vi "Main.vi"() -> ()   [LabVIEW 2016]
uses:
  <vilib>/picture/picture.llb/imagedata.ctl
panel:
  out "nInterfaceNum":u32
  in  "Path":path
  in  "SavePic":bool
  in  "pConvertInfo In 2":T1
  out "frameHandle":i64
  in  "DeviceInterfaceType":u16(ring) items=["GigE", "U3v", "CameraLink", "CXP"]
  in  "ExposureAuto":i32(ring)
  out "QuitFlag":bool
  in  "pConvertInfo In":T1
  in  "image data":T2 caption="图像数据"
  in  "Rectangle":T3
  in  "DeviceScanType":i32(ring)
  out "InterfaceOpened":bool
  out "hDev":i64
  out "hIFDev":i64
  out "interfaceKeyList":string[](array[string])
  out "HasInterface":bool
  out "Picture":picture
  out "Acquired Frames/s":dbl
  out "Processed Frames/s":dbl
  in  "TriggerSource":i32(ring)
  in  "ExecuteSoftTrig":bool
  in  "CloseTrig":bool
  in  "OpenTrig":bool
  in  "Stop":bool
  in  "Play":bool
  in  "Quit":bool
  in  "Height":i32
  in  "Width":i32
  in  "PixelFormat":i32(ring)
  in  "GainRaw":dbl
  in  "ExposureTime":dbl
  out "IsGrabbing":bool
  out "TrigModeOn":bool
  out "error out":errorcluster
  in  "error in":errorcluster
  in  "Close":bool
  in  "Open":bool
  out "HasDevices":bool
  in  "DeviceOpened":bool
  in  "DeviceList":i64(ring)
  in  "Discovery":bool
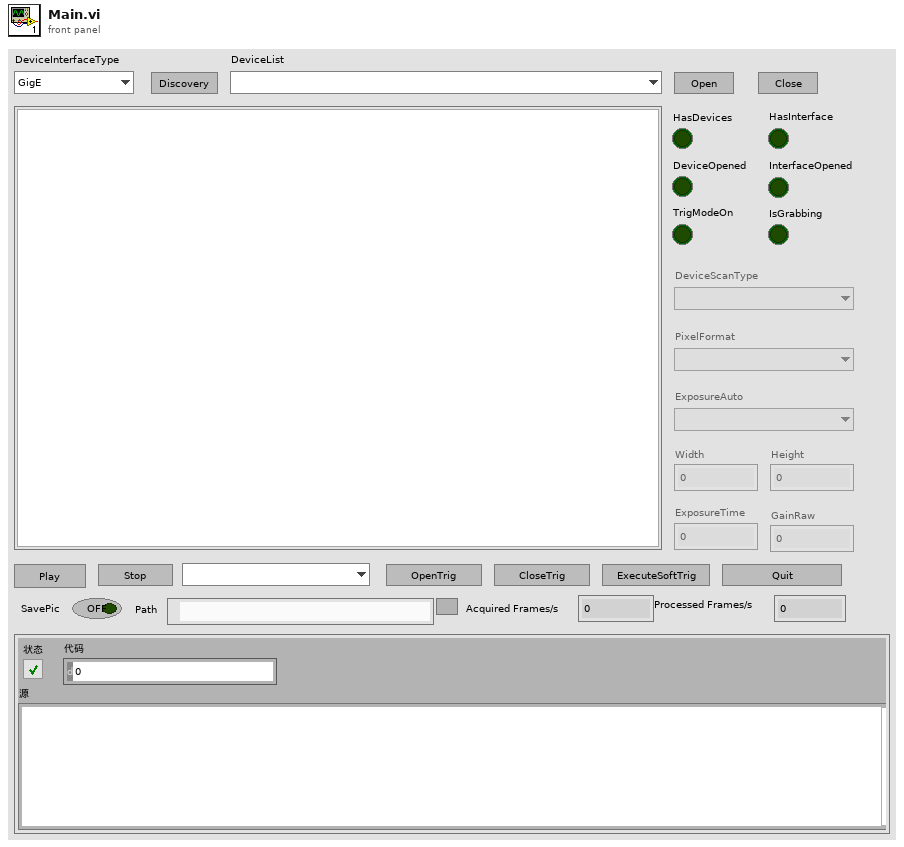
[diagram p1: front panel]
types:
  T1 = cluster{"nWidth":u32, "nHeight":u32, "enSrcPixelType":u32, "nSrcDataLen":u32, "nPaddingX":u32, "nPaddingY":u32, "eBayerDemosaic":u32, "eDstPixelFormat":u32, "nDstBufSize":u32, "nDstDataLen":u32, "nReserved0":u32, "nReserved1":u32, "nReserved2":u32, "nReserved3":u32, "nReserved4":u32, "nReserved5":u32, "nReserved6":u32, "nReserved7":u32}
  T2 = typedef "imagedata.ctl" = cluster{"image type":i32, "image depth":i32, "image":u8[], "mask":u8[], "colors":u32[], "Rectangle":cluster{"left":i16, "top":i16, "right":i16, "bottom":i16}}
  T3 = cluster{"left":i16, "top":i16, "right":i16, "bottom":i16}
  T4 = cluster{"blockId":u64, "status":u32, "width":u32, "height":u32, "size":u32, "pixelFormat":u32, "timeStamp":u64, "chunkCount":u32, "paddingX":u32, "paddingY":u32, "recvFrameTime":u32}
  T5 = cluster{"blockId":u64, "status":u32, "width":u32, "height":u32, "size":u32, "pixelFormat":i32, "timeStamp":u64, "chunkCount":u32, "paddingX":u32, "paddingY":u32, "recvFrameTime":u32}
  T6 = enum8{"Enabled", "Disabled", "Disabled and Grayed Out"}
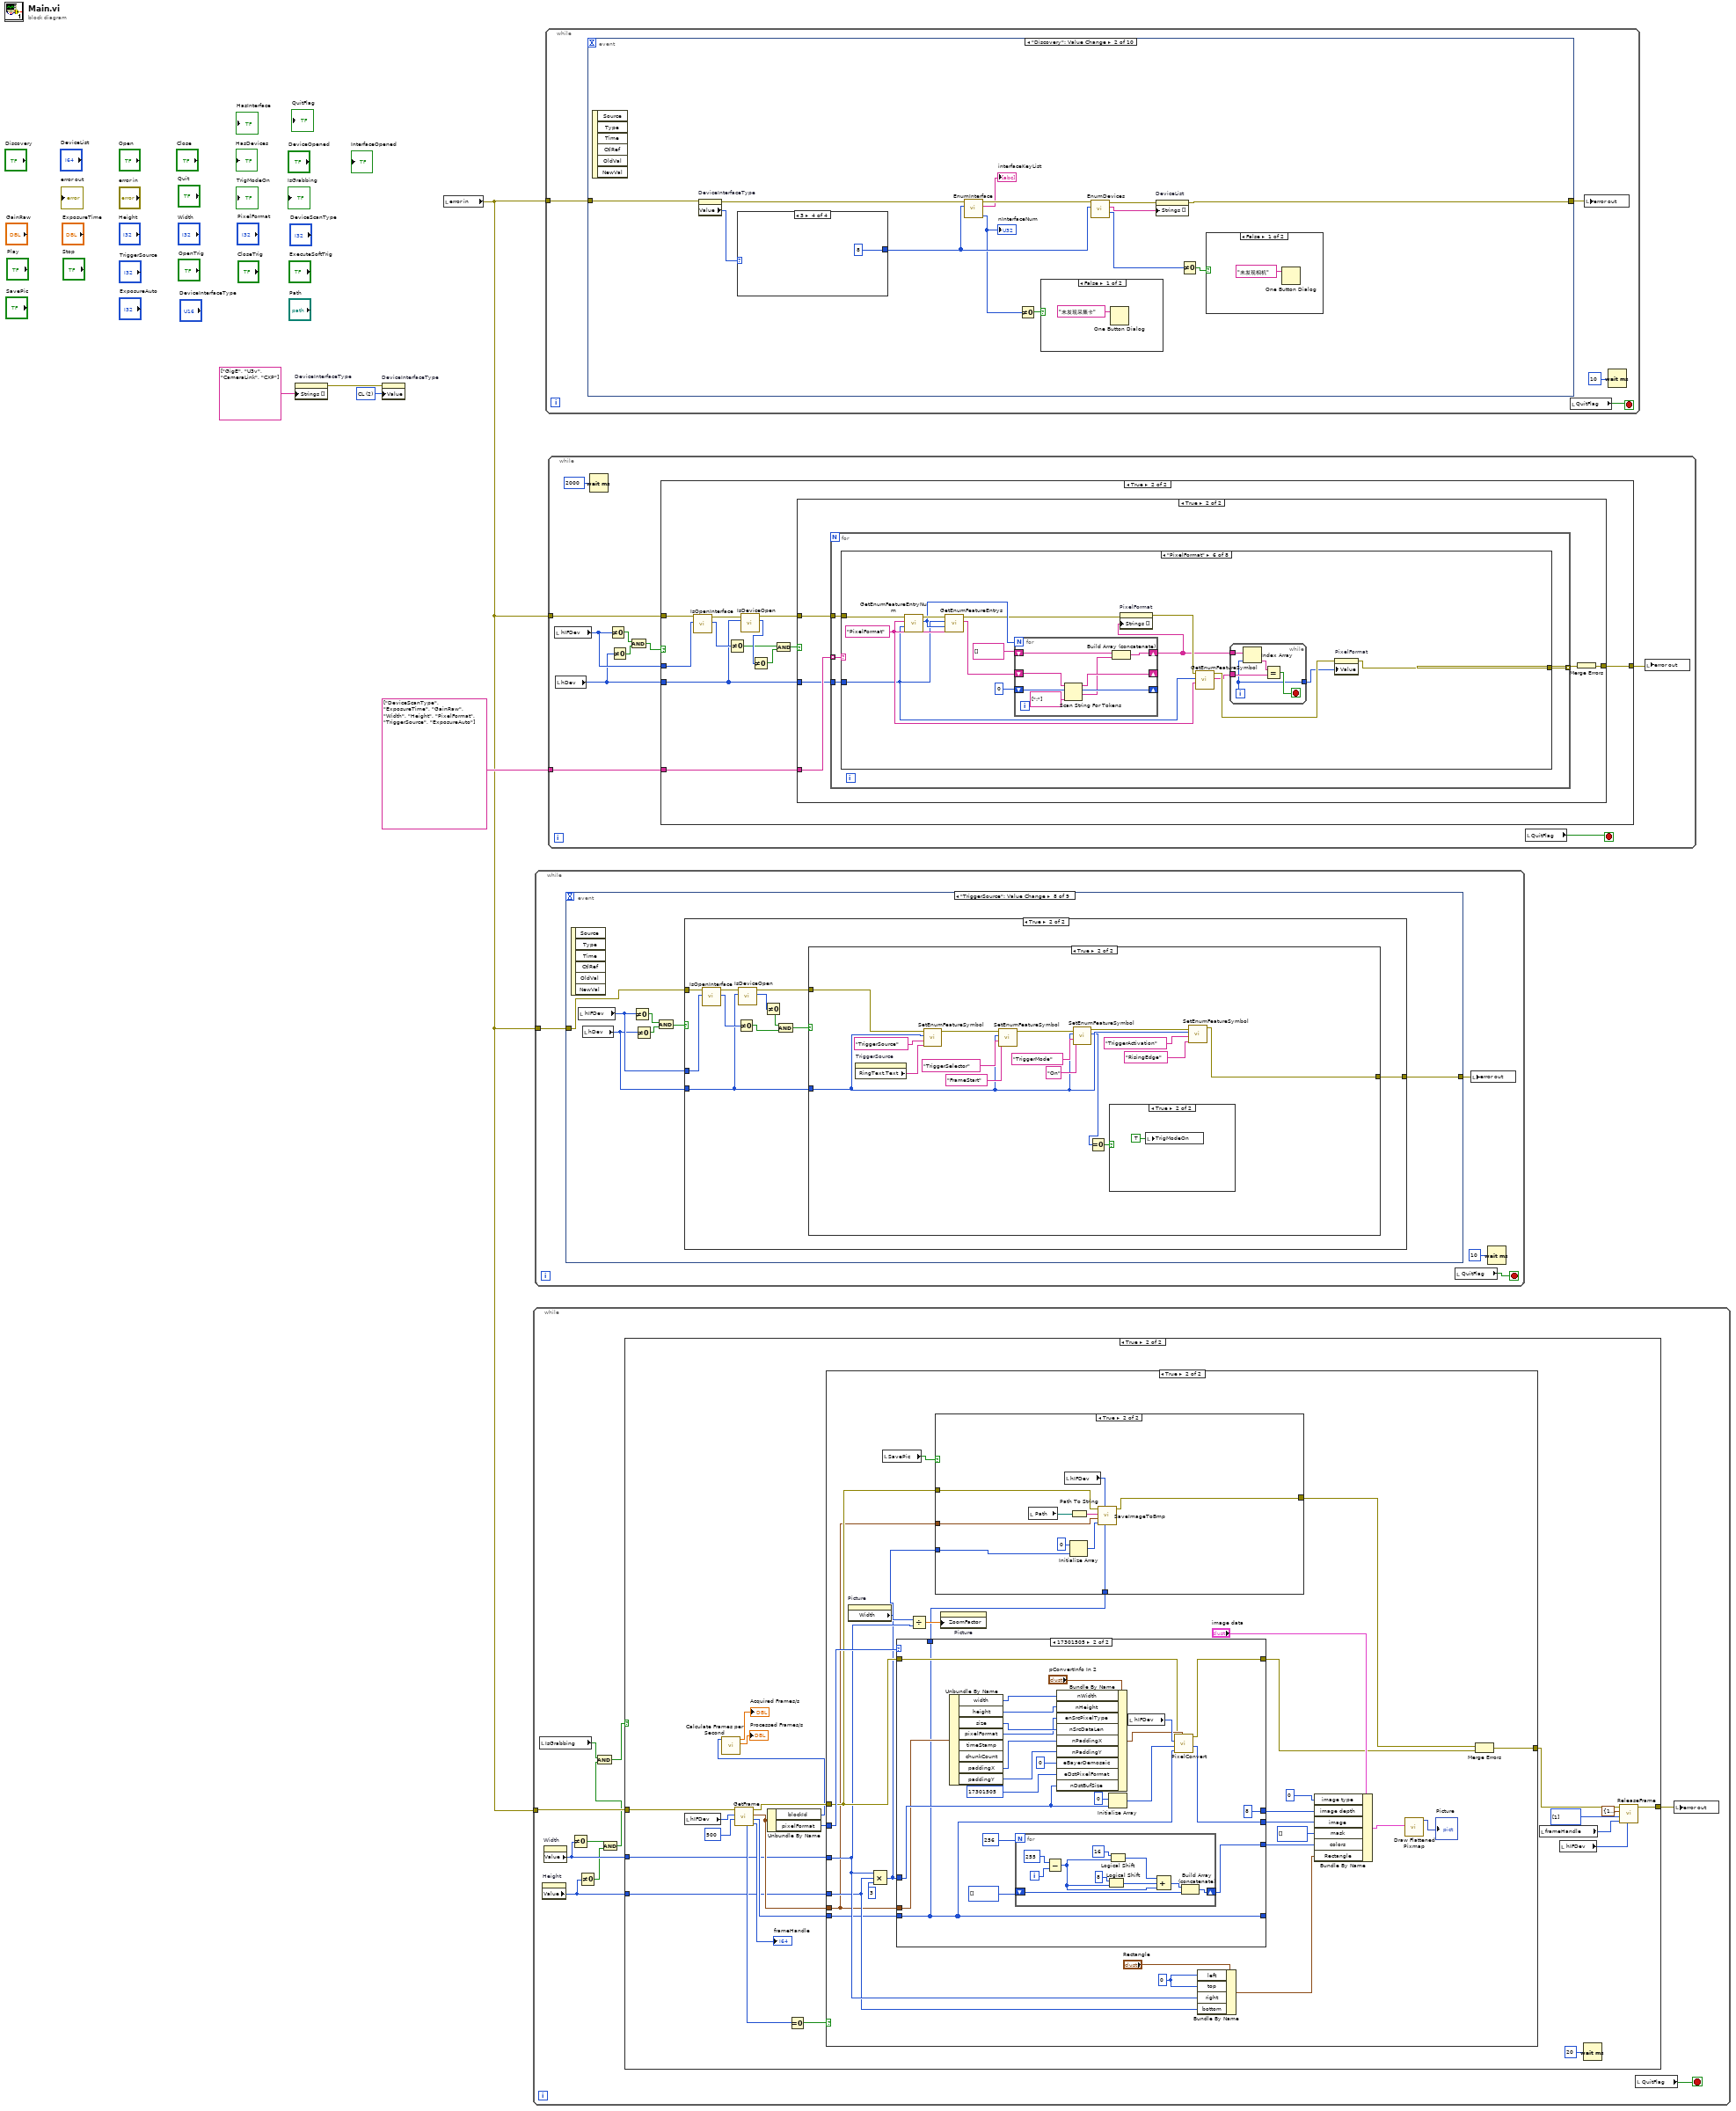
[diagram p0: block diagram]
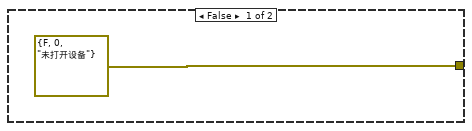
[diagram p2: hidden frame]
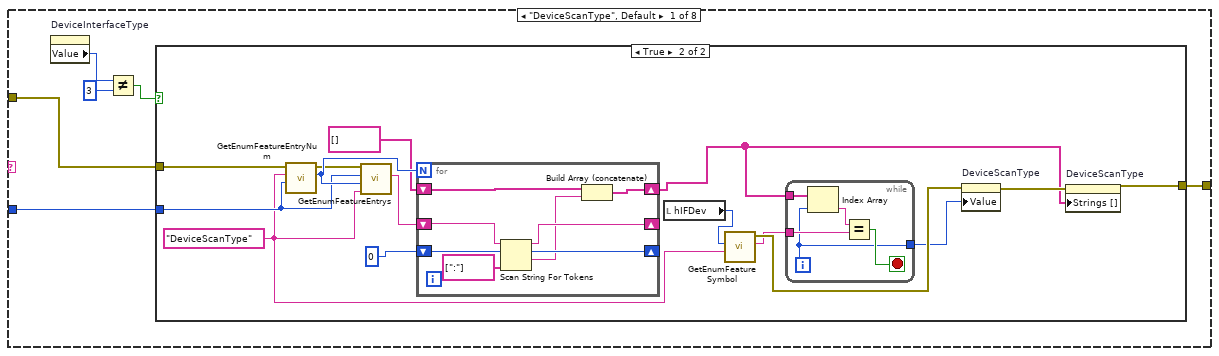
[diagram p4: hidden frame]
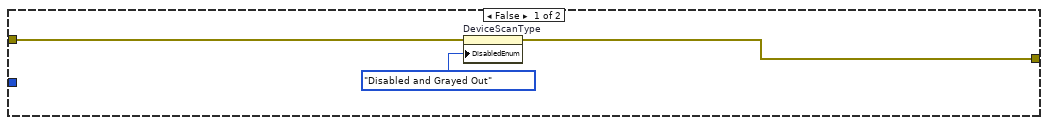
[diagram p5: hidden frame]
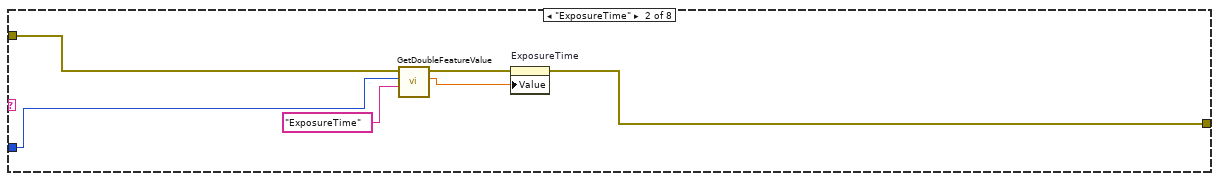
[diagram p6: hidden frame]
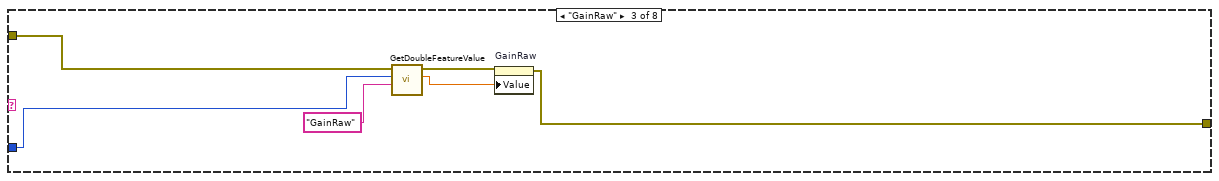
[diagram p7: hidden frame]
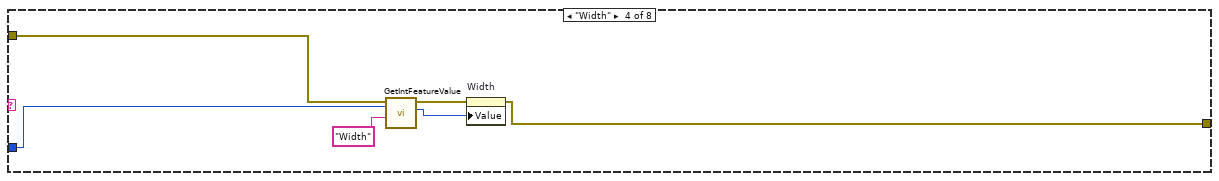
[diagram p8: hidden frame]
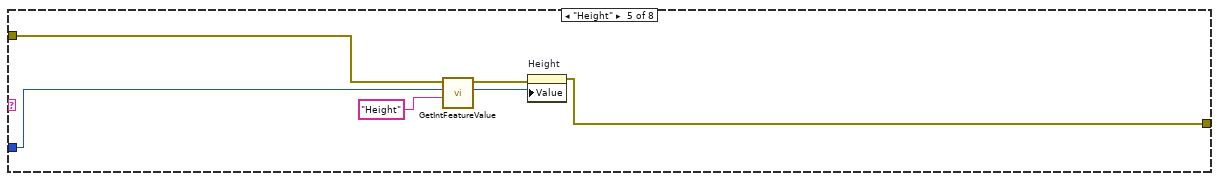
[diagram p9: hidden frame]
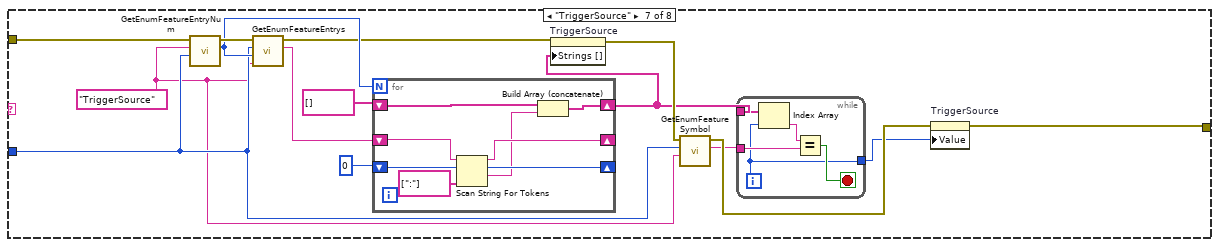
[diagram p10: hidden frame]
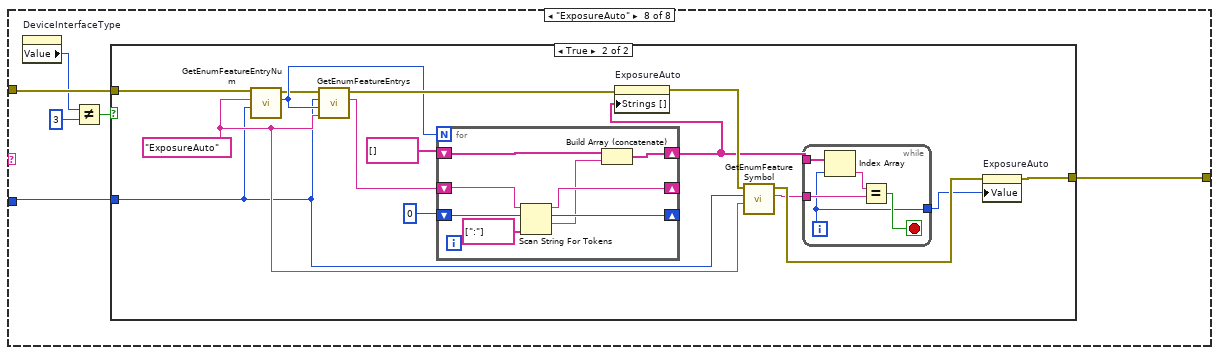
[diagram p11: hidden frame]
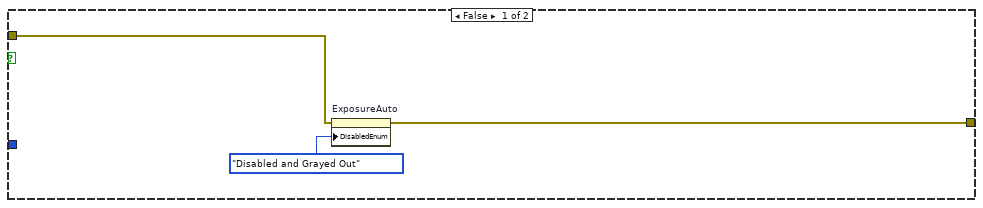
[diagram p12: hidden frame]
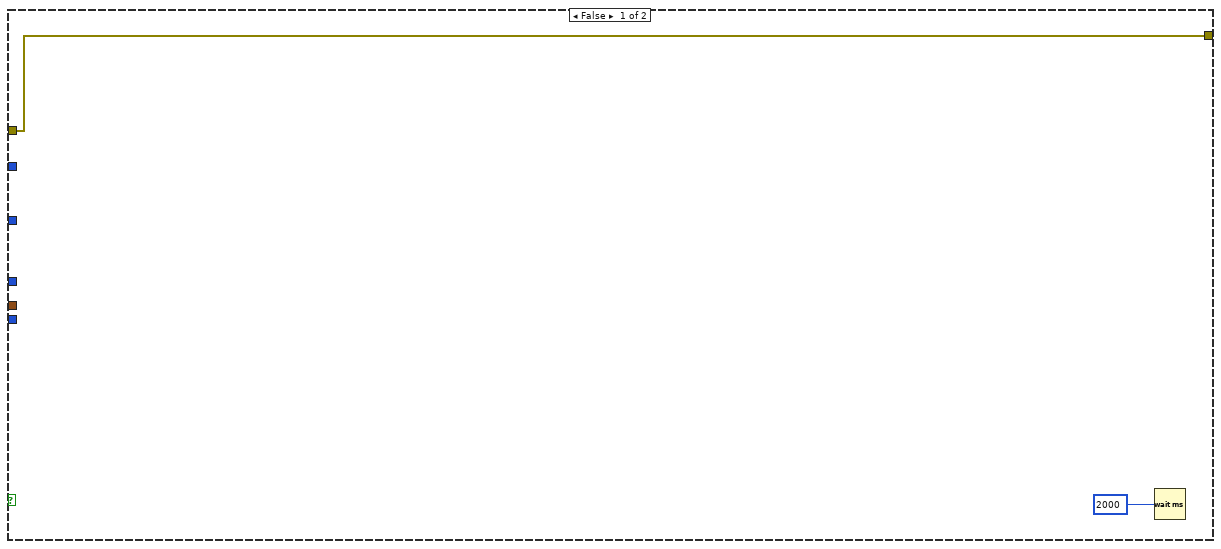
[diagram p14: hidden frame]
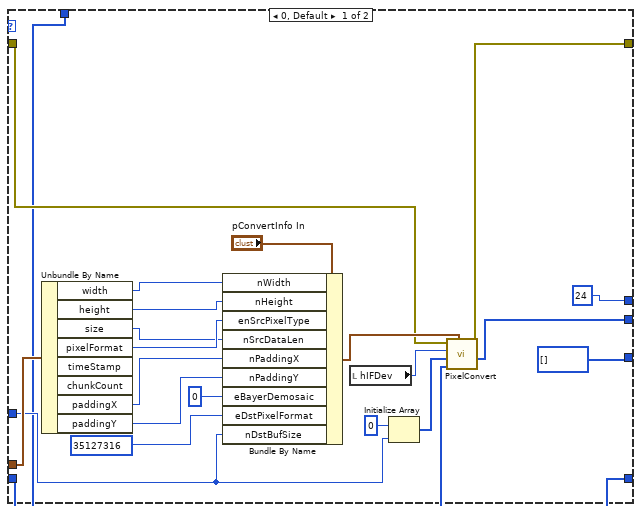
[diagram p16: hidden frame]
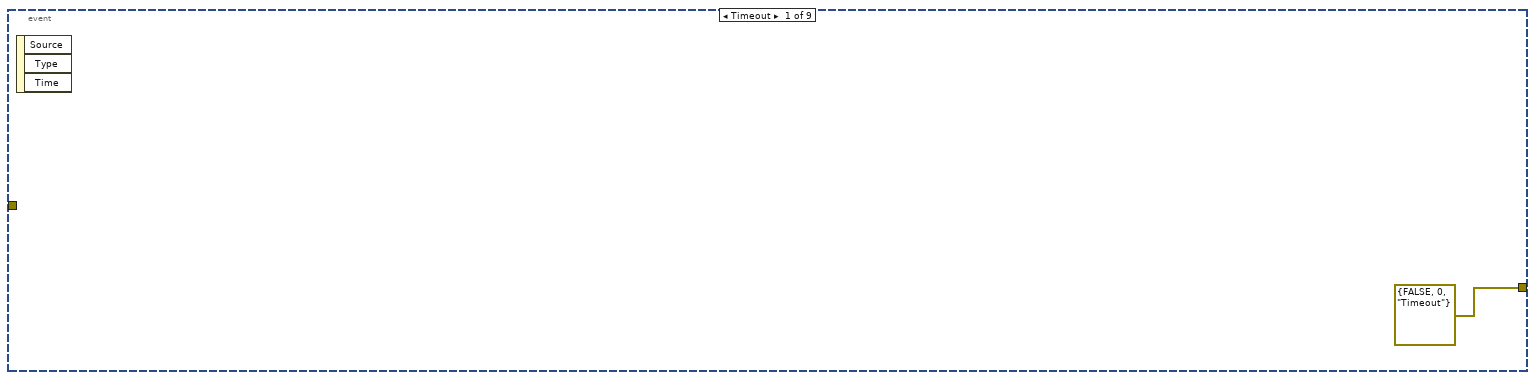
[diagram p17: hidden frame]
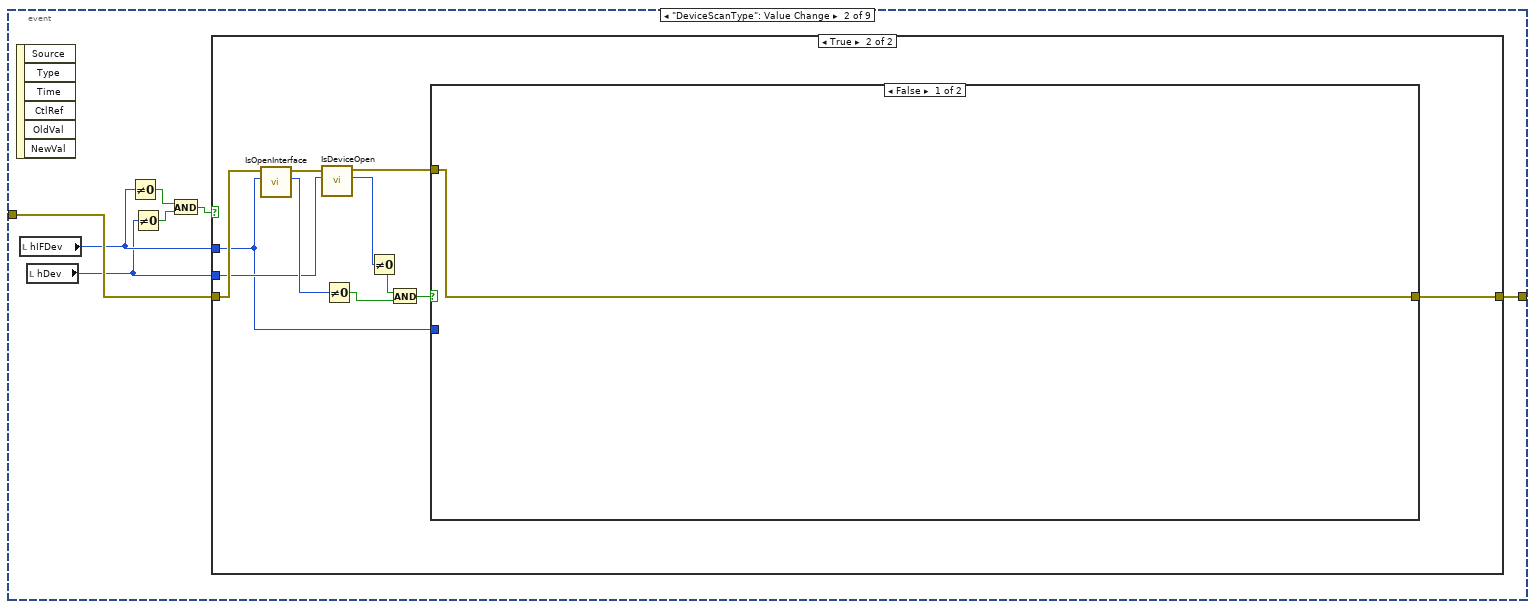
[diagram p18: hidden frame]
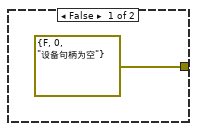
[diagram p19: hidden frame]
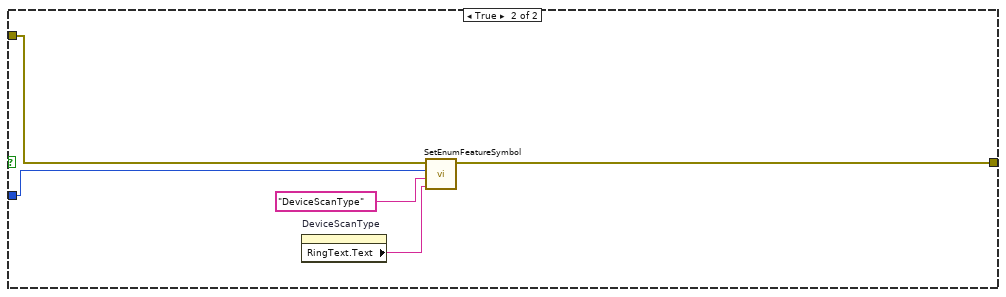
[diagram p20: hidden frame]
diagram:
  w2 = u16 2 items=["GigE", "U3v", "CL", "CXP"] ("DeviceInterfaceType")
  n1 = property on="DeviceInterfaceType" class="Ring (strict)"("Strings []"=string[] ["GigE", "U3v", "CameraLink", "CXP"]) -> (error out=w1:errorcluster)  [unwired: 2 in, 1 out]
  n2 = property on="DeviceInterfaceType" class="Ring (strict)"(error in=w1, "Value"=w2) -> ()  [unwired: 1 in, 2 out]
  n3 = local read "error in"() -> (w4:errorcluster)
  n4 = while {
    tunnel: w4 -> [w15]
    stop <- w13 stop-if-true
    n5 = local read "IsGrabbing"() -> (w8:bool)
    n6 = property on="Height" class="DigNum (strict)"() -> ("Value"=w10:i32)  [unwired: 2 in, 2 out]
    n7 = property on="Width" class="DigNum (strict)"() -> ("Value"=w11:i32)  [unwired: 2 in, 2 out]
    n8 = Not Equal To 0?(x=w11) -> (x != 0?=w12:bool)
    n9 = Not Equal To 0?(x=w10) -> (x != 0?=w9:bool)
    n10 = And(x=w12, y=w9) -> (x .and. y?=w7:bool)
    n11 = And(x=w8, y=w7) -> (x .and. y?=w6:bool)
    n12 = case shown="True" w6 {
      tunnel: w15 -> [w16 w24]
      tunnel: [w16 w28] -> w14
      tunnel: w11 -> [_ w20]
      tunnel: w10 -> [_ w19]
      frame False {
      }
      frame True {
        n13 = local read "hIFDev"() -> (w22:i64)
        n14 = call "GetFrame.vi"("timeoutMS"=u32 500, "handle"=w22, "error in (no error)"=w24) -> ("frameHandle"=→"frameHandle":i64, "pData"=w35:u8[], "pLbFrame out"=w36:T5, "error out"=w30:errorcluster, "return type"=w38:i32)  [unwired: 4 in]
        n15 = Unbundle By Name(w36) -> ("blockId"=w27:u64, "pixelFormat"=w31:i32)
        n16 = call <vilib>:"Calculate Frames per Second.vi"("Buffer Number"=w27) -> ("Processed Frames/s"=→"Processed Frames/s":dbl, "Acquired Frames/s"=→"Acquired Frames/s":dbl)  [unwired: 8 in, 1 out]
        n17 = Equal To 0?(x=w38) -> (x = 0?=w37:bool)
        n18 = case shown="True" w37 {
          tunnel: w36 -> [_ w45]
          tunnel: w35 -> [_ w43]
          tunnel: w20 -> [_ w47]
          tunnel: w19 -> [_ w46]
          tunnel: w31 -> [_ w63]
          tunnel: w30 -> [w40 w52]
          tunnel: [w40 w49] -> w29
          frame False {
            n19 = Wait (ms)(milliseconds to wait=u32 2000 ("等待时间（毫秒）")) -> ()  [unwired: 1 out]
          }
          frame True {
            w61 = i16 0 ("left")
            n20 = property on="Picture" class="Pict"() -> ("Width"=w65:u32)  [unwired: 2 in, 2 out]
            n21 = Compound Arithmetic op=MULTIPLY(w47, w46, 3) -> (w44:i32)
            n22 = local read "SavePic"() -> (w42:bool)
            n23 = case shown="17301505" w63 {
              tunnel: [i32[] [] w119] -> w56
              tunnel: w43 -> [w78 w99]
              tunnel: [w78 w99] -> _
              tunnel: [w86 w100] -> w53
              tunnel: [24 8] -> w54
              tunnel: w45 -> [w81 w106]
              tunnel: w52 -> [w83 w102]
              tunnel: [w82 w101] -> w50
              tunnel: w44 -> [w80 w107]
              tunnel: [w78 w99] -> w41
              frame 0, Default {
                n24 = Unbundle By Name(w81) -> ("width"=w97:u32, "height"=w96:u32, "size"=w79:u32, "pixelFormat"=w95:i32, "paddingX"=w94:u32, "paddingY"=w93:u32)  [unwired: 2 out]
                n25 = Bundle By Name(cluster="pConvertInfo In", "nWidth"=w97, "nHeight"=w96, "enSrcPixelType"=w95, "nSrcDataLen"=w79, "nPaddingX"=w94, "nPaddingY"=w93, "eBayerDemosaic"=u32 0, "eDstPixelFormat"=u32 35127316 ("enDstPixelType"), "nDstBufSize"=w80) -> (w89:T1)
                n26 = local read "hIFDev"() -> (w88:i64)
                n27 = Initialize Array(u8 0, w80) -> (w87:u8[])
                n28 = call "PixelConvert.vi"("lbPstPixelConvertParam"=w89, "pSrcData"=w78, "pDstBuf"=w87, "Interface handle"=w88, "error in (no error)"=w83) -> ("pDstBuf out"=w86:u8[], "error out"=w82:errorcluster)  [unwired: 5 in]
              }
              frame 17301505 {
                n29 = Unbundle By Name(w106) -> ("width"=w110:u32, "height"=w111:u32, "size"=w117:u32, "pixelFormat"=w112:i32, "paddingX"=w113:u32, "paddingY"=w114:u32)  [unwired: 2 out]
                n30 = for {
                  N: 256 -> [_]
                  shift-right: [w126] -> w119
                  shift-left: i32[] [] ("数组") -> [w125]
                  i -> [w122]
                  n31 = Subtract(x=255, y=w122) -> (x-y=w123:i32)
                  n32 = Logical Shift(y=i16 8, x=w123) -> (x << y=w128:i32)
                  n33 = Logical Shift(y=16 ("x"), x=w123) -> (x << y=w129:i32)
                  n34 = Compound Arithmetic op=ADD(w129, w128, w123) -> (w127:i32)
                  n35 = Build Array (concatenate)(w127, w125) -> (w126:i32[])
                }
                n36 = Bundle By Name(cluster="pConvertInfo In 2", "nWidth"=w110, "nHeight"=w111, "enSrcPixelType"=w112, "nSrcDataLen"=w117, "nPaddingX"=w113, "nPaddingY"=w114, "eBayerDemosaic"=u32 0, "eDstPixelFormat"=u32 17301505 ("enDstPixelType"), "nDstBufSize"=w107) -> (w103:T1)
                n37 = Initialize Array(u8 0, w107) -> (w104:u8[])
                n38 = local read "hIFDev"() -> (w105:i64)
                n39 = call "PixelConvert.vi"("lbPstPixelConvertParam"=w103, "pSrcData"=w99, "pDstBuf"=w104, "Interface handle"=w105, "error in (no error)"=w102) -> ("pDstBuf out"=w100:u8[], "error out"=w101:errorcluster)  [unwired: 5 in]
              }
            }
            n40 = Divide(x=w65, y=w47) -> (x/y=w64:dbl)
            n41 = case shown="True" w42 {
              tunnel: w52 -> [w67 w77]
              tunnel: [w67 w76] -> w51
              tunnel: w45 -> [_ w75]
              tunnel: w44 -> [_ w74]
              tunnel: w41 -> [_ w73]
              frame False {
              }
              frame True {
                n42 = local read "Path"() -> (w72:path)
                n43 = local read "hIFDev"() -> (w70:i64)
                n44 = Initialize Array(u8 0, w74) -> (w68:u8[])
                n45 = Path To String(path=w72) -> (string=w71:string)
                n46 = call "SaveImageToBmp.vi"("pSrcData"=w73, "interface handle"=w70, "pDstBuf"=w68, "pLbFrame"=w75, "filePath"=w71, "error in (no error)"=w77) -> ("error out"=w76:errorcluster)  [unwired: 4 in, 1 out]
              }
            }
            n47 = property on="Picture" class="Pict"("ZoomFactor"=w64) -> ()  [unwired: 2 in, 2 out]
            n48 = Bundle By Name(cluster="Rectangle", "left"=w61, "top"=w61, "right"=w47, "bottom"=w46) -> (w57:T3)
            n49 = Bundle By Name(cluster="image data", "image type"=0, "image depth"=w54, "image"=w53, "mask"=u8[] [], "colors"=w56, "Rectangle"=w57) -> (w59:T2)
            n50 = call <vilib>:"Draw Flattened Pixmap.vi"("image data"=w59) -> ("new picture"=→"Picture":picture)  [unwired: 8 in]
            n51 = Merge Errors(w51, w50) -> (w49:errorcluster)
          }
        }
        n52 = local read "frameHandle"() -> (w23:i64)
        n53 = local read "hIFDev"() -> (w33:i64)
        n54 = Wait (ms)(milliseconds to wait=u32 20 ("等待时间（毫秒）")) -> ()  [unwired: 1 out]
        n55 = call "ReleaseFrame.vi"("interface handle"=w33, "frameHandle"=w23, "pData"=u8[] [1], "pLbFrame"=T4 {"blockId"=1, "status"=0, "width"=0, "height"=0, "size"=0, "pixelFormat"=0, "timeStamp"=0, "chunkCount"=0, "paddingX"=0, "paddingY"=0, "recvFrameTime"=0}, "error in (no error)"=w29) -> ("error out"=w28:errorcluster)  [unwired: 6 in]
      }
    }
    n56 = local read "QuitFlag"() -> (w13:bool)
    n57 = local write "error out"(w14) -> ()
  }
  n58 = while {
    tunnel: w4 -> [w135]
    stop <- w133 stop-if-true
    n59 = event shown="[7] \"TriggerSource\": Value Change" {
      selector: _ -> [_ _ _ _ _ _ _ _ _]
      dyn-events: _ -> [_ _ _ _ _ _ _ _ _]
      timeout: _ -> [_ _ _ _ _ _ _ _ _]
      tunnel: w135 -> [_ w143 w167 w192 w217 w244 w271 w293 w330]
      tunnel: [errorcluster {FALSE, 0, "Timeout"} w142 w168 w193 w218 w245 w272 w294 w331] -> w134
      event Timeout {
        n60 = event-data() -> ()  [unwired: 1 in, 3 out]
      }
      event "DeviceScanType": Value Change {
        n61 = event-data() -> ()  [unwired: 1 in, 6 out]
        n62 = local read "hIFDev"() -> (w138:i64)
        n63 = local read "hDev"() -> (w137:i64)
        n64 = Not Equal To 0?(x=w138) -> (x != 0?=w141:bool)
        n65 = Not Equal To 0?(x=w137) -> (x != 0?=w140:bool)
        n66 = And(x=w141, y=w140) -> (x .and. y?=w139:bool)
        n67 = case shown="True" w139 {
          tunnel: w143 -> [_ w155]
          tunnel: [errorcluster {"status"=FALSE, "code"=0, "source"="设备句柄为空"} ("error in") w147] -> w142
          tunnel: w138 -> [_ w145]
          tunnel: w137 -> [_ w146]
          frame False {
          }
          frame True {
            n68 = call "IsOpenInterface.vi"("interface handle"=w145, "error in (no error)"=w155) -> ("return type"=w151:i8, "error out"=w154:errorcluster)  [unwired: 8 in]
            n69 = call "IsDeviceOpen.vi"("dev handle"=w146, "error in (no error)"=w154) -> ("return type"=w152:i8, "error out"=w153:errorcluster)  [unwired: 8 in]
            n70 = Not Equal To 0?(x=w151) -> (x != 0?=w148:bool)
            n71 = Not Equal To 0?(x=w152) -> (x != 0?=w149:bool)
            n72 = And(x=w149, y=w148) -> (x .and. y?=w150:bool)
            n73 = case shown="False" w150 {
              tunnel: w153 -> [w156 w161]
              tunnel: [w156 w160] -> w147
              tunnel: w145 -> [_ w157]
              frame False {
              }
              frame True {
                n74 = property on="DeviceScanType" class="Ring (strict)"() -> ("RingText.Text"=w158:string)  [unwired: 2 in, 2 out]
                n75 = call "SetEnumFeatureSymbol.vi"("pEnumSymbol"=w158, "pFeatureName"="DeviceScanType", "handle"=w157, "error in (no error)"=w161) -> ("error out"=w160:errorcluster)  [unwired: 6 in, 1 out]
              }
            }
          }
        }
      }
      event "ExposureTime": Value Change {
        n76 = event-data() -> ()  [unwired: 1 in, 6 out]
        n77 = local read "hDev"() -> (w165:i64)
        n78 = local read "hIFDev"() -> (w166:i64)
        n79 = Not Equal To 0?(x=w166) -> (x != 0?=w164:bool)
        n80 = Not Equal To 0?(x=w165) -> (x != 0?=w163:bool)
        n81 = And(x=w164, y=w163) -> (x .and. y?=w162:bool)
        n82 = case shown="True" w162 {
          tunnel: [errorcluster {FALSE, 0, "设备句柄为空"} w171] -> w168
          tunnel: w166 -> [_ w175]
          tunnel: w165 -> [_ w172]
          tunnel: w167 -> [_ w170]
          frame False {
          }
          frame True {
            n83 = call "IsOpenInterface.vi"("interface handle"=w175, "error in (no error)"=w170) -> ("return type"=w178:i8, "error out"=w176:errorcluster)  [unwired: 8 in]
            n84 = Not Equal To 0?(x=w178) -> (x != 0?=w180:bool)
            n85 = call "IsDeviceOpen.vi"("dev handle"=w172, "error in (no error)"=w176) -> ("return type"=w177:i8, "error out"=w173:errorcluster)  [unwired: 8 in]
            n86 = Not Equal To 0?(x=w177) -> (x != 0?=w179:bool)
            n87 = And(x=w179, y=w180) -> (x .and. y?=w174:bool)
            n88 = case shown="True" w174 {
              tunnel: w173 -> [w181 w186]
              tunnel: w172 -> [_ w185]
              tunnel: [w181 w182] -> w171
              frame False {
              }
              frame True {
                n89 = property on="ExposureTime" class="DigNum (strict)"() -> ("Value"=w183:dbl)  [unwired: 2 in, 2 out]
                n90 = call "SetDoubleFeatureValue.vi"("doubleValue"=w183, "pFeatureName"="ExposureTime", "handle"=w185, "error in (no error)"=w186) -> ("error out"=w182:errorcluster)  [unwired: 7 in]
              }
            }
          }
        }
      }
      event "GainRaw": Value Change {
        n91 = event-data() -> ()  [unwired: 1 in, 6 out]
        n92 = local read "hIFDev"() -> (w190:i64)
        n93 = local read "hDev"() -> (w189:i64)
        n94 = Not Equal To 0?(x=w190) -> (x != 0?=w187:bool)
        n95 = Not Equal To 0?(x=w189) -> (x != 0?=w188:bool)
        n96 = And(x=w187, y=w188) -> (x .and. y?=w191:bool)
        n97 = case shown="True" w191 {
          tunnel: w190 -> [_ w199]
          tunnel: w189 -> [_ w196]
          tunnel: [errorcluster {FALSE, 0, "设备句柄为空"} w197] -> w193
          tunnel: w192 -> [_ w195]
          frame False {
          }
          frame True {
            n98 = call "IsOpenInterface.vi"("interface handle"=w199, "error in (no error)"=w195) -> ("return type"=w203:i8, "error out"=w201:errorcluster)  [unwired: 8 in]
            n99 = Not Equal To 0?(x=w203) -> (x != 0?=w205:bool)
            n100 = call "IsDeviceOpen.vi"("dev handle"=w196, "error in (no error)"=w201) -> ("return type"=w202:i8, "error out"=w198:errorcluster)  [unwired: 8 in]
            n101 = Not Equal To 0?(x=w202) -> (x != 0?=w204:bool)
            n102 = And(x=w204, y=w205) -> (x .and. y?=w200:bool)
            n103 = case shown="True" w200 {
              tunnel: w198 -> [w206 w211]
              tunnel: [w206 w207] -> w197
              tunnel: w196 -> [_ w210]
              frame False {
              }
              frame True {
                n104 = property on="GainRaw" class="DigNum (strict)"() -> ("Value"=w208:dbl)  [unwired: 2 in, 2 out]
                n105 = call "SetDoubleFeatureValue.vi"("doubleValue"=w208, "pFeatureName"="GainRaw", "handle"=w210, "error in (no error)"=w211) -> ("error out"=w207:errorcluster)  [unwired: 7 in]
              }
            }
          }
        }
      }
      event "Width": Value Change {
        n106 = event-data() -> ()  [unwired: 1 in, 6 out]
        n107 = local read "hIFDev"() -> (w215:i64)
        n108 = local read "hDev"() -> (w214:i64)
        n109 = Not Equal To 0?(x=w215) -> (x != 0?=w213:bool)
        n110 = Not Equal To 0?(x=w214) -> (x != 0?=w212:bool)
        n111 = And(x=w213, y=w212) -> (x .and. y?=w216:bool)
        n112 = case shown="True" w216 {
          tunnel: [errorcluster {"status"=FALSE, "code"=0, "source"="设备句柄为空"} ("error in") w224] -> w218
          tunnel: w215 -> [_ w220]
          tunnel: w214 -> [_ w222]
          tunnel: w217 -> [_ w221]
          frame False {
          }
          frame True {
            n113 = call "IsOpenInterface.vi"("interface handle"=w220, "error in (no error)"=w221) -> ("return type"=w228:i8, "error out"=w230:errorcluster)  [unwired: 8 in]
            n114 = Not Equal To 0?(x=w228) -> (x != 0?=w226:bool)
            n115 = call "IsDeviceOpen.vi"("dev handle"=w222, "error in (no error)"=w230) -> ("return type"=w229:i8, "error out"=w225:errorcluster)  [unwired: 8 in]
            n116 = Not Equal To 0?(x=w229) -> (x != 0?=w227:bool)
            n117 = And(x=w227, y=w226) -> (x .and. y?=w223:bool)
            n118 = case shown="True" w223 {
              tunnel: w225 -> [w231 w237]
              tunnel: [w231 w235] -> w224
              tunnel: w222 -> [_ w238]
              tunnel: w220 -> [_ w234]
              frame False {
              }
              frame True {
                w233 = "Width" ("pFeatureName")
                n119 = property on="Width" class="DigNum (strict)"() -> ("Value"=w232:i32)  [unwired: 2 in, 2 out]
                n120 = call "SetIntFeatureValue.vi"("intValue"=w232, "pFeatureName"=w233, "handle"=w238, "error in (no error)"=w237) -> ("error out"=w236:errorcluster)  [unwired: 7 in]
                n121 = call "SetIntFeatureValue.vi"("intValue"=w232, "pFeatureName"=w233, "handle"=w234, "error in (no error)"=w236) -> ("error out"=w235:errorcluster)  [unwired: 7 in]
              }
            }
          }
        }
      }
      event "Height": Value Change {
        n122 = event-data() -> ()  [unwired: 1 in, 6 out]
        n123 = local read "hIFDev"() -> (w240:i64)
        n124 = local read "hDev"() -> (w239:i64)
        n125 = Not Equal To 0?(x=w240) -> (x != 0?=w242:bool)
        n126 = Not Equal To 0?(x=w239) -> (x != 0?=w241:bool)
        n127 = And(x=w242, y=w241) -> (x .and. y?=w243:bool)
        n128 = case shown="True" w243 {
          tunnel: [errorcluster {FALSE, 0, "设备句柄为空"} w250] -> w245
          tunnel: w240 -> [_ w247]
          tunnel: w239 -> [_ w249]
          tunnel: w244 -> [_ w248]
          frame False {
          }
          frame True {
            n129 = call "IsOpenInterface.vi"("interface handle"=w247, "error in (no error)"=w248) -> ("return type"=w255:i8, "error out"=w253:errorcluster)  [unwired: 8 in]
            n130 = Not Equal To 0?(x=w255) -> (x != 0?=w257:bool)
            n131 = call "IsDeviceOpen.vi"("dev handle"=w249, "error in (no error)"=w253) -> ("return type"=w254:i8, "error out"=w251:errorcluster)  [unwired: 8 in]
            n132 = Not Equal To 0?(x=w254) -> (x != 0?=w256:bool)
            n133 = And(x=w256, y=w257) -> (x .and. y?=w252:bool)
            n134 = case shown="True" w252 {
              tunnel: w251 -> [w258 w265]
              tunnel: [w258 w259] -> w250
              tunnel: w249 -> [_ w264]
              tunnel: w247 -> [_ w260]
              frame False {
              }
              frame True {
                w262 = "Height" ("pFeatureName")
                n135 = property on="Height" class="DigNum (strict)"() -> ("Value"=w261:i32)  [unwired: 2 in, 2 out]
                n136 = call "SetIntFeatureValue.vi"("intValue"=w261, "pFeatureName"=w262, "handle"=w264, "error in (no error)"=w265) -> ("error out"=w263:errorcluster)  [unwired: 7 in]
                n137 = call "SetIntFeatureValue.vi"("intValue"=w261, "pFeatureName"=w262, "handle"=w260, "error in (no error)"=w263) -> ("error out"=w259:errorcluster)  [unwired: 7 in]
              }
            }
          }
        }
      }
      event "PixelFormat": Value Change {
        n138 = event-data() -> ()  [unwired: 1 in, 6 out]
        n139 = local read "hIFDev"() -> (w269:i64)
        n140 = local read "hDev"() -> (w268:i64)
        n141 = Not Equal To 0?(x=w269) -> (x != 0?=w266:bool)
        n142 = Not Equal To 0?(x=w268) -> (x != 0?=w267:bool)
        n143 = And(x=w266, y=w267) -> (x .and. y?=w270:bool)
        n144 = case shown="True" w270 {
          tunnel: [errorcluster {FALSE, 0, "设备句柄为空"} w277] -> w272
          tunnel: w269 -> [_ w274]
          tunnel: w268 -> [_ w276]
          tunnel: w271 -> [_ w275]
          frame False {
          }
          frame True {
            n145 = call "IsOpenInterface.vi"("interface handle"=w274, "error in (no error)"=w275) -> ("return type"=w283:i8, "error out"=w280:errorcluster)  [unwired: 8 in]
            n146 = Not Equal To 0?(x=w283) -> (x != 0?=w281:bool)
            n147 = call "IsDeviceOpen.vi"("dev handle"=w276, "error in (no error)"=w280) -> ("return type"=w284:i8, "error out"=w278:errorcluster)  [unwired: 8 in]
            n148 = Not Equal To 0?(x=w284) -> (x != 0?=w282:bool)
            n149 = And(x=w282, y=w281) -> (x .and. y?=w279:bool)
            n150 = case shown="True" w279 {
              tunnel: w278 -> [w285 w292]
              tunnel: [w285 w286] -> w277
              tunnel: w276 -> [_ w291]
              tunnel: w274 -> [_ w287]
              frame False {
              }
              frame True {
                w289 = "PixelFormat" ("pFeatureName")
                n151 = property on="PixelFormat" class="Ring (strict)"() -> ("RingText.Text"=w288:string)  [unwired: 2 in, 2 out]
                n152 = call "SetEnumFeatureSymbol.vi"("pEnumSymbol"=w288, "pFeatureName"=w289, "handle"=w291, "error in (no error)"=w292) -> ("error out"=w290:errorcluster)  [unwired: 6 in, 1 out]
                n153 = call "SetEnumFeatureSymbol.vi"("pEnumSymbol"=w288, "pFeatureName"=w289, "handle"=w287, "error in (no error)"=w290) -> ("error out"=w286:errorcluster)  [unwired: 6 in, 1 out]
              }
            }
          }
        }
      }
      event "TriggerSource": Value Change {
        n154 = event-data() -> ()  [unwired: 1 in, 6 out]
        n155 = local read "hIFDev"() -> (w296:i64)
        n156 = local read "hDev"() -> (w295:i64)
        n157 = Not Equal To 0?(x=w296) -> (x != 0?=w299:bool)
        n158 = Not Equal To 0?(x=w295) -> (x != 0?=w298:bool)
        n159 = And(x=w299, y=w298) -> (x .and. y?=w297:bool)
        n160 = case shown="True" w297 {
          tunnel: w296 -> [_ w307]
          tunnel: w295 -> [_ w302]
          tunnel: [errorcluster {"status"=FALSE, "code"=0, "source"="设备句柄为空"} ("error in") w301] -> w294
          tunnel: w293 -> [_ w305]
          frame False {
          }
          frame True {
            n161 = call "IsOpenInterface.vi"("interface handle"=w307, "error in (no error)"=w305) -> ("return type"=w309:i8, "error out"=w304:errorcluster)  [unwired: 8 in]
            n162 = Not Equal To 0?(x=w309) -> (x != 0?=w311:bool)
            n163 = call "IsDeviceOpen.vi"("dev handle"=w302, "error in (no error)"=w304) -> ("return type"=w308:i8, "error out"=w303:errorcluster)  [unwired: 8 in]
            n164 = Not Equal To 0?(x=w308) -> (x != 0?=w310:bool)
            n165 = And(x=w310, y=w311) -> (x .and. y?=w306:bool)
            n166 = case shown="True" w306 {
              tunnel: w303 -> [w312 w328]
              tunnel: w302 -> [_ w318]
              tunnel: [w312 w315] -> w301
              frame False {
              }
              frame True {
                n167 = property on="TriggerSource" class="Ring (strict)"() -> ("RingText.Text"=w326:string)  [unwired: 2 in, 2 out]
                n168 = call "SetEnumFeatureSymbol.vi"("pEnumSymbol"=w326, "pFeatureName"="TriggerSource", "handle"=w318, "error in (no error)"=w328) -> ("error out"=w325:errorcluster)  [unwired: 6 in, 1 out]
                n169 = call "SetEnumFeatureSymbol.vi"("pEnumSymbol"="FrameStart", "pFeatureName"="TriggerSelector", "handle"=w318, "error in (no error)"=w325) -> ("error out"=w322:errorcluster)  [unwired: 6 in, 1 out]
                n170 = call "SetEnumFeatureSymbol.vi"("pEnumSymbol"="On", "pFeatureName"="TriggerMode", "handle"=w318, "error in (no error)"=w322) -> ("return type"=w313:i32, "error out"=w321:errorcluster)  [unwired: 6 in]
                n171 = Equal To 0?(x=w313) -> (x = 0?=w314:bool)
                n172 = case shown="True" w314 {
                  frame False {
                  }
                  frame True {
                    n173 = local write "TrigModeOn"(TRUE ("TrigModeOn")) -> ()
                  }
                }
                n174 = call "SetEnumFeatureSymbol.vi"("pEnumSymbol"="RisingEdge", "pFeatureName"="TriggerActivation", "handle"=w318, "error in (no error)"=w321) -> ("error out"=w315:errorcluster)  [unwired: 6 in, 1 out]
              }
            }
          }
        }
      }
      event "ExposureAuto": Value Change {
        n175 = event-data() -> ()  [unwired: 1 in, 6 out]
        n176 = local read "hIFDev"() -> (w333:i64)
        n177 = local read "hDev"() -> (w332:i64)
        n178 = Not Equal To 0?(x=w333) -> (x != 0?=w335:bool)
        n179 = Not Equal To 0?(x=w332) -> (x != 0?=w336:bool)
        n180 = And(x=w335, y=w336) -> (x .and. y?=w334:bool)
        n181 = case shown="True" w334 {
          tunnel: w333 -> [_ w342]
          tunnel: w332 -> [_ w338]
          tunnel: [errorcluster {"status"=FALSE, "code"=0, "source"="设备句柄为空"} ("error in") w339] -> w331
          tunnel: w330 -> [_ w343]
          frame False {
          }
          frame True {
            n182 = call "IsOpenInterface.vi"("interface handle"=w342, "error in (no error)"=w343) -> ("return type"=w346:i8, "error out"=w348:errorcluster)  [unwired: 8 in]
            n183 = Not Equal To 0?(x=w346) -> (x != 0?=w344:bool)
            n184 = call "IsDeviceOpen.vi"("dev handle"=w338, "error in (no error)"=w348) -> ("return type"=w347:i8, "error out"=w340:errorcluster)  [unwired: 8 in]
            n185 = Not Equal To 0?(x=w347) -> (x != 0?=w345:bool)
            n186 = And(x=w345, y=w344) -> (x .and. y?=w341:bool)
            n187 = case shown="True" w341 {
              tunnel: [w349 w353] -> w339
              tunnel: w340 -> [w349 w354]
              tunnel: w338 -> [_ w352]
              frame False {
              }
              frame True {
                n188 = property on="ExposureAuto" class="Ring (strict)"() -> ("RingText.Text"=w350:string)  [unwired: 2 in, 2 out]
                n189 = call "SetEnumFeatureSymbol.vi"("pEnumSymbol"=w350, "pFeatureName"="ExposureAuto", "handle"=w352, "error in (no error)"=w354) -> ("error out"=w353:errorcluster)  [unwired: 6 in, 1 out]
              }
            }
          }
        }
      }
    }
    n190 = local read "QuitFlag"() -> (w133:bool)
    n191 = local write "error out"(w134) -> ()
    n192 = Wait (ms)(milliseconds to wait=u32 10 ("等待时间（毫秒）")) -> ()  [unwired: 1 out]
  }
  n193 = while {
    tunnel: w4 -> [w357]
    stop <- w356 stop-if-true
    n194 = event shown="[1] \"Discovery\": Value Change" {
      selector: _ -> [_ _ _ _ _ _ _ _ _ _]
      dyn-events: _ -> [_ _ _ _ _ _ _ _ _ _]
      timeout: _ -> [_ _ _ _ _ _ _ _ _ _]
      tunnel: [errorcluster {FALSE, 0, "Timeout"} w364 w382 w420 w446 w495 w514 w532 w538 w543] -> w358
      tunnel: w357 -> [_ w365 w407 w441 w447 w511 w513 w534 w541 w544]
      event Timeout {
        n195 = event-data() -> ()  [unwired: 1 in, 3 out]
      }
      event "Discovery": Value Change {
        n196 = event-data() -> ()  [unwired: 1 in, 6 out]
        n197 = property on="DeviceInterfaceType" class="Ring (strict)"(error in=w365) -> (error out=w368:errorcluster, "Value"=w367:u16)  [unwired: 1 in, 1 out]
        n198 = case shown="3" w367 {
          tunnel: [u32 1 u32 2 u32 4 u32 8] -> w366
          frame 0, Default {
          }
          frame 1 {
          }
          frame 2 {
          }
          frame 3 {
          }
        }
        n199 = call "EnumInterface.vi"("nInterfaceType"=w366, "error in"=w368) -> ("nInterfaceNum"=w362:u32, "interfaceKeyList"=→"interfaceKeyList":string[], "error out"=w370:errorcluster)  [unwired: 7 in]
        "nInterfaceNum" <- w362
        n200 = Not Equal To 0?(x=w362) -> (x != 0?=w363:bool)
        n201 = case shown="False" w363 {
          frame False {
            n202 = One Button Dialog(message="未发现采集卡") -> ()  [unwired: 1 in, 1 out]
          }
          frame True {
            n203 = local write "HasInterface"(TRUE ("HasInterface")) -> ()
          }
        }
        n204 = call "EnumDevices.vi"("nDeviceType"=w366, "error in"=w370) -> ("nDeviceNum"=w361:i32, "deviceKeyList"=w371:string[], "error out"=w372:errorcluster)  [unwired: 7 in]
        n205 = property on="DeviceList" class="Ring (strict)"(error in=w372, "Strings []"=w371) -> (error out=w364:errorcluster)  [unwired: 1 in, 1 out]
        n206 = Not Equal To 0?(x=w361) -> (x != 0?=w360:bool)
        n207 = case shown="False" w360 {
          frame False {
            n208 = One Button Dialog(message="未发现相机") -> ()  [unwired: 1 in, 1 out]
          }
          frame True {
            n209 = local write "HasDevices"(TRUE ("HasDevices")) -> ()
          }
        }
      }
      event "Open": Value Change {
        (unwired) T6."Enabled" ("Disabled")
        n210 = event-data() -> ()  [unwired: 1 in, 6 out]
        n211 = local read "nInterfaceNum"() -> (w405:u32)
        n212 = local read "interfaceKeyList"() -> (w406:string[])
        n213 = while {
          tunnel: w406 -> [w419]
          tunnel: [w417] -> w381
          tunnel: w405 -> [w410]
          i -> [w417]
          stop <- w414 stop-if-true
          n214 = property on="DeviceList" class="Ring (strict)"() -> ("RingText.Text"=w413:string)  [unwired: 2 in, 2 out]
          n215 = Index Array(array=w419, index=w417) -> (element=w418:string)
          n216 = Search/Split String(string=w413, search string/char (-)="[") -> (substring before match=w411:string)  [unwired: 1 in, 2 out]
          n217 = Equal?(x=w418, y=w411) -> (x = y?=w416:bool)
          n218 = Greater Or Equal?(x=w417, y=w410) -> (x >= y?=w415:bool)
          n219 = Or(x=w416, y=w415) -> (x .or. y?=w414:bool)
        }
        n220 = call "OpenInterface.vi"("nIndex"=w381, "error in (no error)"=w407) -> ("hIFDev"=w401:i64, "error out"=w404:errorcluster)  [unwired: 7 in, 1 out]
        "hIFDev" <- w401
        n221 = property on="DeviceList" class="Ring (strict)"() -> ("Value"=w402:i64)  [unwired: 2 in, 2 out]
        n222 = Not Equal To 0?(x=w401) -> (x != 0?=w398:bool)
        n223 = call "OpenDevice.vi"("pIdentifier"=w402, "mode"=0, "error in (no error)"=w404) -> ("hDev"=w400:i64, "error out"=w383:errorcluster)  [unwired: 6 in, 1 out]
        "hDev" <- w400
        n224 = Not Equal To 0?(x=w400) -> (x != 0?=w399:bool)
        n225 = And(x=w399, y=w398) -> (x .and. y?=w397:bool)
        n226 = case shown="True" w397 {
          frame False {
          }
          frame True {
            n227 = local write "DeviceOpened"(TRUE ("DeviceOpened")) -> ()
            n228 = local write "InterfaceOpened"(TRUE ("InterfaceOpened")) -> ()
          }
        }
        n229 = property on="DeviceScanType" class="Ring (strict)"(error in=w383, "DisabledEnum"=T6."Enabled" ("Disabled")) -> (error out=w386:errorcluster)  [unwired: 1 in, 1 out]
        n230 = property on="GainRaw" class="DigNum (strict)"(error in=w386, "DisabledEnum"=T6."Enabled" ("Disabled")) -> (error out=w384:errorcluster)  [unwired: 1 in, 1 out]
        n231 = property on="Width" class="DigNum (strict)"(error in=w384, "DisabledEnum"=T6."Enabled" ("Disabled")) -> (error out=w392:errorcluster)  [unwired: 1 in, 1 out]
        n232 = property on="Height" class="DigNum (strict)"(error in=w392, "DisabledEnum"=T6."Enabled" ("Disabled")) -> (error out=w387:errorcluster)  [unwired: 1 in, 1 out]
        n233 = property on="ExposureTime" class="DigNum (strict)"(error in=w387, "DisabledEnum"=T6."Enabled" ("Disabled")) -> (error out=w393:errorcluster)  [unwired: 1 in, 1 out]
        n234 = property on="PixelFormat" class="Ring (strict)"(error in=w393, "DisabledEnum"=T6."Enabled" ("Disabled")) -> (error out=w395:errorcluster)  [unwired: 1 in, 1 out]
        n235 = property on="ExposureAuto" class="Ring (strict)"(error in=w395, "DisabledEnum"=T6."Enabled" ("Disabled")) -> (error out=w382:errorcluster)  [unwired: 1 in, 1 out]
      }
      event "Close": Value Change {
        (unwired) T6."Disabled and Grayed Out" ("Disabled")
        n236 = event-data() -> ()  [unwired: 1 in, 6 out]
        n237 = local read "hDev"() -> (w440:i64)
        n238 = call "CloseDevice.vi"("dev handle"=w440, "error in (no error)"=w441) -> ("return type"=w437:i32, "error out"=w439:errorcluster)  [unwired: 8 in]
        n239 = local read "hIFDev"() -> (w438:i64)
        n240 = call "CloseInterface.vi"("interface handle"=w438, "error in (no error)"=w439) -> ("return type"=w435:i32, "error out"=w421:errorcluster)  [unwired: 8 in]
        n241 = Equal To 0?(x=w437) -> (x = 0?=w436:bool)
        n242 = case shown="True" w436 {
          tunnel: w435 -> [_ w444]
          frame False {
          }
          frame True {
            n243 = Equal To 0?(x=w444) -> (x = 0?=w443:bool)
            n244 = local write "DeviceOpened"(FALSE ("DeviceOpened")) -> ()
            n245 = case shown="True" w443 {
              frame False {
              }
              frame True {
                n246 = local write "InterfaceOpened"(FALSE ("InterfaceOpened")) -> ()
              }
            }
          }
        }
        n247 = property on="DeviceScanType" class="Ring (strict)"(error in=w421, "DisabledEnum"=T6."Disabled and Grayed Out" ("Disabled")) -> (error out=w424:errorcluster)  [unwired: 1 in, 1 out]
        n248 = property on="ExposureTime" class="DigNum (strict)"(error in=w424, "DisabledEnum"=T6."Disabled and Grayed Out" ("Disabled")) -> (error out=w422:errorcluster)  [unwired: 1 in, 1 out]
        n249 = property on="PixelFormat" class="Ring (strict)"(error in=w422, "DisabledEnum"=T6."Disabled and Grayed Out" ("Disabled")) -> (error out=w430:errorcluster)  [unwired: 1 in, 1 out]
        n250 = property on="Width" class="DigNum (strict)"(error in=w430, "DisabledEnum"=T6."Disabled and Grayed Out" ("Disabled")) -> (error out=w425:errorcluster)  [unwired: 1 in, 1 out]
        n251 = property on="Height" class="DigNum (strict)"(error in=w425, "DisabledEnum"=T6."Disabled and Grayed Out" ("Disabled")) -> (error out=w431:errorcluster)  [unwired: 1 in, 1 out]
        n252 = property on="GainRaw" class="DigNum (strict)"(error in=w431, "DisabledEnum"=T6."Disabled and Grayed Out" ("Disabled")) -> (error out=w433:errorcluster)  [unwired: 1 in, 1 out]
        n253 = property on="ExposureAuto" class="Ring (strict)"(error in=w433, "DisabledEnum"=T6."Disabled and Grayed Out" ("Disabled")) -> (error out=w420:errorcluster)  [unwired: 1 in, 1 out]
      }
      event "Play": Value Change {
        n254 = event-data() -> ()  [unwired: 1 in, 6 out]
        n255 = local read "hIFDev"() -> (w449:i64)
        n256 = local read "hDev"() -> (w448:i64)
        n257 = Not Equal To 0?(x=w449) -> (x != 0?=w451:bool)
        n258 = Not Equal To 0?(x=w448) -> (x != 0?=w452:bool)
        n259 = And(x=w451, y=w452) -> (x .and. y?=w450:bool)
        n260 = case shown="True" w450 {
          tunnel: w449 -> [_ w455]
          tunnel: w448 -> [_ w458]
          tunnel: w447 -> [_ w456]
          tunnel: [errorcluster {"status"=FALSE, "code"=0, "source"="未打开相机"} ("error out") w454] -> w446
          frame False {
          }
          frame True {
            n261 = call "IsOpenInterface.vi"("interface handle"=w455) -> ("return type"=w462:i8)  [unwired: 9 in, 1 out]
            n262 = Not Equal To 0?(x=w462) -> (x != 0?=w461:bool)
            n263 = call "IsDeviceOpen.vi"("dev handle"=w458) -> ("return type"=w459:i8)  [unwired: 9 in, 1 out]
            n264 = Not Equal To 0?(x=w459) -> (x != 0?=w460:bool)
            n265 = And(x=w461, y=w460) -> (x .and. y?=w457:bool)
            n266 = case shown="True" w457 {
              tunnel: w456 -> [_ w467]
              tunnel: w455 -> [_ w466]
              tunnel: [errorcluster {"status"=FALSE, "code"=0, "source"="未打开相机"} ("error out") w469] -> w454
              frame False {
              }
              frame True {
                n267 = call "IsGrabbing.vi"("interface handle"=w466, "error in (no error)"=w467) -> ("return type"=w464:i8, "error out"=w468:errorcluster)  [unwired: 8 in]
                n268 = Equal To 0?(x=w464) -> (x = 0?=w465:bool)
                n269 = case shown="True" w465 {
                  tunnel: [w470 w477] -> w469
                  tunnel: w468 -> [w470 w474]
                  tunnel: w466 -> [_ w473]
                  frame False {
                  }
                  frame True {
                    n270 = call "SetBufferCount.vi"("nSize"=u32 2, "interface handle"=w473, "error in (no error)"=w474) -> ("error out"=w476:errorcluster)  [unwired: 7 in, 1 out]
                    n271 = call "StartGrabbing.vi"("interface handle"=w473, "error in (no error)"=w476) -> ("return type"=w471:i32, "error out"=w480:errorcluster)  [unwired: 8 in]
                    n272 = Equal To 0?(x=w471) -> (x = 0?=w472:bool)
                    n273 = case shown="True" w472 {
                      frame False {
                      }
                      frame True {
                        n274 = local write "IsGrabbing"(TRUE ("IsGrabbing")) -> ()
                      }
                    }
                    n275 = property on="ExposureAuto" class="Ring (strict)"(error in=w480, "DisabledEnum"=T6."Enabled" ("Disabled")) -> (error out=w479:errorcluster)  [unwired: 1 in, 1 out]
                    n276 = property on="DeviceScanType" class="Ring (strict)"(error in=w479, "DisabledEnum"=T6."Enabled" ("Disabled")) -> (error out=w487:errorcluster)  [unwired: 1 in, 1 out]
                    n277 = property on="ExposureTime" class="DigNum (strict)"(error in=w487, "DisabledEnum"=T6."Enabled" ("Disabled")) -> (error out=w488:errorcluster)  [unwired: 1 in, 1 out]
                    n278 = property on="GainRaw" class="DigNum (strict)"(error in=w488, "DisabledEnum"=T6."Enabled" ("Disabled")) -> (error out=w489:errorcluster)  [unwired: 1 in, 1 out]
                    n279 = property on="Width" class="DigNum (strict)"(error in=w489, "DisabledEnum"=T6."Disabled and Grayed Out" ("Disabled")) -> (error out=w490:errorcluster)  [unwired: 1 in, 1 out]
                    n280 = property on="Height" class="DigNum (strict)"(error in=w490, "DisabledEnum"=T6."Disabled and Grayed Out" ("Disabled")) -> (error out=w491:errorcluster)  [unwired: 1 in, 1 out]
                    n281 = property on="PixelFormat" class="Ring (strict)"(error in=w491, "DisabledEnum"=T6."Disabled and Grayed Out" ("Disabled")) -> (error out=w477:errorcluster)  [unwired: 1 in, 1 out]
                  }
                }
              }
            }
          }
        }
      }
      event "Stop": Value Change {
        n282 = event-data() -> ()  [unwired: 1 in, 6 out]
        n283 = local read "hIFDev"() -> (w510:i64)
        n284 = call "StopGrabbing.vi"("interface handle"=w510, "error in (no error)"=w511) -> ("return type"=w493:i32, "error out"=w503:errorcluster)  [unwired: 8 in]
        n285 = Equal To 0?(x=w493) -> (x = 0?=w494:bool)
        n286 = case shown="True" w494 {
          frame False {
          }
          frame True {
            n287 = local write "IsGrabbing"(FALSE ("IsGrabbing")) -> ()
          }
        }
        n288 = property on="DeviceScanType" class="Ring (strict)"(error in=w503, "DisabledEnum"=T6."Enabled" ("Disabled")) -> (error out=w502:errorcluster)  [unwired: 1 in, 1 out]
        n289 = property on="ExposureTime" class="DigNum (strict)"(error in=w502, "DisabledEnum"=T6."Enabled" ("Disabled")) -> (error out=w501:errorcluster)  [unwired: 1 in, 1 out]
        n290 = property on="GainRaw" class="DigNum (strict)"(error in=w501, "DisabledEnum"=T6."Enabled" ("Disabled")) -> (error out=w500:errorcluster)  [unwired: 1 in, 1 out]
        n291 = property on="Width" class="DigNum (strict)"(error in=w500, "DisabledEnum"=T6."Enabled" ("Disabled")) -> (error out=w499:errorcluster)  [unwired: 1 in, 1 out]
        n292 = property on="Height" class="DigNum (strict)"(error in=w499, "DisabledEnum"=T6."Enabled" ("Disabled")) -> (error out=w498:errorcluster)  [unwired: 1 in, 1 out]
        n293 = property on="PixelFormat" class="Ring (strict)"(error in=w498, "DisabledEnum"=T6."Enabled" ("Disabled")) -> (error out=w497:errorcluster)  [unwired: 1 in, 1 out]
        n294 = property on="ExposureAuto" class="Ring (strict)"(error in=w497, "DisabledEnum"=T6."Enabled" ("Disabled")) -> (error out=w495:errorcluster)  [unwired: 1 in, 1 out]
      }
      event "OpenTrig": Value Change {
        n295 = event-data() -> ()  [unwired: 1 in, 6 out]
        n296 = local read "hDev"() -> (w517:i64)
        n297 = call "SetEnumFeatureSymbol.vi"("pEnumSymbol"="Software", "pFeatureName"="TriggerSource", "handle"=w517, "error in (no error)"=w513) -> ("error out"=w526:errorcluster)  [unwired: 6 in, 1 out]
        n298 = call "SetDoubleFeatureValue.vi"("doubleValue"=0.0, "pFeatureName"="LineDebouncerTime", "handle"=w517, "error in (no error)"=w526) -> ("error out"=w523:errorcluster)  [unwired: 7 in]
        n299 = call "SetEnumFeatureSymbol.vi"("pEnumSymbol"="CC1", "pFeatureName"="LineSelector", "handle"=w517, "error in (no error)"=w523) -> ("error out"=w520:errorcluster)  [unwired: 6 in, 1 out]
        n300 = call "SetEnumFeatureSymbol.vi"("pEnumSymbol"="On", "pFeatureName"="TriggerMode", "handle"=w517, "error in (no error)"=w520) -> ("return type"=w516:i32, "error out"=w514:errorcluster)  [unwired: 6 in]
        n301 = Equal To 0?(x=w516) -> (x = 0?=w515:bool)
        n302 = case shown="True" w515 {
          frame False {
          }
          frame True {
            n303 = local write "TrigModeOn"(TRUE ("TrigModeOn")) -> ()
          }
        }
      }
      event "CloseTrig": Value Change {
        n304 = event-data() -> ()  [unwired: 1 in, 6 out]
        n305 = local read "hDev"() -> (w530:i64)
        n306 = call "SetEnumFeatureSymbol.vi"("pEnumSymbol"="Off", "pFeatureName"="TriggerMode", "handle"=w530, "error in (no error)"=w534) -> ("return type"=w533:i32, "error out"=w532:errorcluster)  [unwired: 6 in]
        n307 = Equal To 0?(x=w533) -> (x = 0?=w531:bool)
        n308 = case shown="True" w531 {
          frame False {
          }
          frame True {
            n309 = local write "TrigModeOn"(FALSE ("TrigModeOn")) -> ()
          }
        }
      }
      event "ExecuteSoftTrig": Value Change {
        n310 = event-data() -> ()  [unwired: 1 in, 6 out]
        n311 = local read "hDev"() -> (w540:i64)
        n312 = call "ExecuteCommandFeature.vi"("pFeatureName"="TriggerSoftware", "handle"=w540, "error in (no error)"=w541) -> ("error out"=w538:errorcluster)  [unwired: 7 in, 1 out]
      }
      event "Quit": Value Change {
        n313 = event-data() -> ()  [unwired: 1 in, 6 out]
        n314 = flat-sequence {
          tunnel: w544 -> [w547]
          tunnel: [w547] -> w542
          tunnel: [w560] -> w543
          tunnel: w542 -> [w579]
          frame #0 {
            n315 = local write "SavePic"(FALSE ("SavePic")) -> ()
            n316 = Wait (ms)(milliseconds to wait=u32 500 ("等待时间（毫秒）")) -> ()  [unwired: 1 out]
          }
          frame #1 {
            (unwired) T6."Disabled and Grayed Out" ("Disabled")
            n317 = local read "hDev"() -> (w563:i64)
            n318 = call "SetEnumFeatureSymbol.vi"("pEnumSymbol"="Off", "pFeatureName"="TriggerMode", "handle"=w563, "error in (no error)"=w579) -> ("return type"=w578:i32, "error out"=w576:errorcluster)  [unwired: 6 in]
            n319 = local read "hIFDev"() -> (w562:i64)
            n320 = Equal To 0?(x=w578) -> (x = 0?=w577:bool)
            n321 = case shown="True" w577 {
              frame False {
              }
              frame True {
                n322 = local write "TrigModeOn"(FALSE ("TrigModeOn")) -> ()
              }
            }
            n323 = call "StopGrabbing.vi"("interface handle"=w562, "error in (no error)"=w576) -> ("return type"=w548:i32, "error out"=w553:errorcluster)  [unwired: 8 in]
            n324 = Equal To 0?(x=w548) -> (x = 0?=w549:bool)
            n325 = case shown="True" w549 {
              frame False {
              }
              frame True {
                n326 = local write "IsGrabbing"(FALSE ("IsGrabbing")) -> ()
              }
            }
            n327 = property on="ExposureAuto" class="Ring (strict)"(error in=w553, "DisabledEnum"=T6."Disabled and Grayed Out" ("Disabled")) -> (error out=w552:errorcluster)  [unwired: 1 in, 1 out]
            n328 = property on="DeviceScanType" class="Ring (strict)"(error in=w552, "DisabledEnum"=T6."Disabled and Grayed Out" ("Disabled")) -> (error out=w573:errorcluster)  [unwired: 1 in, 1 out]
            n329 = property on="PixelFormat" class="Ring (strict)"(error in=w573, "DisabledEnum"=T6."Disabled and Grayed Out" ("Disabled")) -> (error out=w575:errorcluster)  [unwired: 1 in, 1 out]
            n330 = local write "HasInterface"(FALSE ("HasInterface")) -> ()
            n331 = property on="Height" class="DigNum (strict)"(error in=w575, "DisabledEnum"=T6."Disabled and Grayed Out" ("Disabled")) -> (error out=w567:errorcluster)  [unwired: 1 in, 1 out]
            n332 = local write "QuitFlag"(FALSE ("QuitFlag")) -> ()
            n333 = local write "HasDevices"(FALSE ("HasDevices")) -> ()
            n334 = property on="Width" class="DigNum (strict)"(error in=w567, "DisabledEnum"=T6."Disabled and Grayed Out" ("Disabled")) -> (error out=w572:errorcluster)  [unwired: 1 in, 1 out]
            n335 = property on="ExposureTime" class="DigNum (strict)"(error in=w572, "DisabledEnum"=T6."Disabled and Grayed Out" ("Disabled")) -> (error out=w566:errorcluster)  [unwired: 1 in, 1 out]
            n336 = property on="GainRaw" class="DigNum (strict)"(error in=w566, "DisabledEnum"=T6."Disabled and Grayed Out" ("Disabled")) -> (error out=w564:errorcluster)  [unwired: 1 in, 1 out]
            n337 = property on="DeviceList" class="Ring (strict)"("Strings []"=string[] []) -> ()  [unwired: 2 in, 2 out]
            n338 = call "CloseDevice.vi"("dev handle"=w563, "error in (no error)"=w564) -> ("return type"=w558:i32, "error out"=w561:errorcluster)  [unwired: 8 in]
            n339 = Equal To 0?(x=w558) -> (x = 0?=w559:bool)
            n340 = call "CloseInterface.vi"("interface handle"=w562, "error in (no error)"=w561) -> ("return type"=w557:i32, "error out"=w560:errorcluster)  [unwired: 8 in]
            n341 = case shown="True" w559 {
              tunnel: w557 -> [_ w584]
              frame False {
              }
              frame True {
                n342 = local write "DeviceOpened"(FALSE ("DeviceOpened")) -> ()
                n343 = Equal To 0?(x=w584) -> (x = 0?=w583:bool)
                n344 = case shown="True" w583 {
                  frame False {
                  }
                  frame True {
                    n345 = local write "InterfaceOpened"(FALSE ("InterfaceOpened")) -> ()
                  }
                }
              }
            }
          }
        }
      }
    }
    n346 = local read "QuitFlag"() -> (w356:bool)
    n347 = local write "error out"(w358) -> ()
    n348 = Wait (ms)(milliseconds to wait=u32 10 ("等待时间（毫秒）")) -> ()  [unwired: 1 out]
  }
  n349 = while {
    tunnel: string[] ["DeviceScanType", "ExposureTime", "GainRaw", "Width", "Height", "PixelFormat", "TriggerSource", "ExposureAuto"] -> [w596]
    tunnel: w4 -> [w594]
    stop <- w588 stop-if-true
    n350 = local read "hIFDev"() -> (w593:i64)
    n351 = local read "hDev"() -> (w592:i64)
    n352 = Wait (ms)(milliseconds to wait=u32 2000) -> ()  [unwired: 1 out]
    n353 = Not Equal To 0?(x=w593) -> (x != 0?=w590:bool)
    n354 = Not Equal To 0?(x=w592) -> (x != 0?=w591:bool)
    n355 = And(x=w590, y=w591) -> (x .and. y?=w589:bool)
    n356 = case shown="True" w589 {
      tunnel: w596 -> [_ w610]
      tunnel: w594 -> [_ w608]
      tunnel: [errorcluster {"status"=FALSE, "code"=0, "source"="未打开设备"} ("错误常量") w609] -> w595
      tunnel: w593 -> [_ w600]
      tunnel: w592 -> [_ w599]
      frame False {
      }
      frame True {
        n357 = call "IsOpenInterface.vi"("interface handle"=w600, "error in (no error)"=w608) -> ("return type"=w605:i8, "error out"=w607:errorcluster)  [unwired: 8 in]
        n358 = Not Equal To 0?(x=w605) -> (x != 0?=w603:bool)
        n359 = call "IsDeviceOpen.vi"("dev handle"=w599, "error in (no error)"=w607) -> ("return type"=w604:i8, "error out"=w606:errorcluster)  [unwired: 8 in]
        n360 = Not Equal To 0?(x=w604) -> (x != 0?=w602:bool)
        n361 = And(x=w603, y=w602) -> (x .and. y?=w601:bool)
        n362 = case shown="True" w601 {
          tunnel: w610 -> [_ w616]
          tunnel: [w611 w614] -> w609
          tunnel: w606 -> [w611 w613]
          tunnel: w599 -> [_ w612]
          frame False {
          }
          frame True {
            n363 = for {
              tunnel: w616 -> [w620] mode=indexing
              tunnel: [w619] -> w615 mode=indexing
              tunnel: w613 -> [w618]
              tunnel: w612 -> [w617]
              n364 = case shown="\"PixelFormat\"" w620 {
                tunnel: [w624 w661 w667 w672 w678 w686 w713 w741] -> w619
                tunnel: w618 -> [w626 w659 w665 w671 w677 w696 w717 w743]
                tunnel: w617 -> [w625 w658 w664 w670 w676 w682 w716 w742]
                frame "DeviceScanType", Default {
                  n365 = property on="DeviceInterfaceType" class="Ring (strict)"() -> ("Value"=w622:u16)  [unwired: 2 in, 2 out]
                  n366 = Not Equal?(x=w622, y=3) -> (x != y?=w623:bool)
                  n367 = case shown="True" w623 {
                    tunnel: w626 -> [w627 w638]
                    tunnel: w625 -> [_ w636]
                    tunnel: [w628 w633] -> w624
                    frame False {
                      n368 = property on="DeviceScanType" class="Ring (strict)"(error in=w627, "DisabledEnum"=T6."Disabled and Grayed Out" ("Disabled")) -> (error out=w628:errorcluster)  [unwired: 1 in, 1 out]
                    }
                    frame True {
                      w635 = "DeviceScanType" ("pFeatureName")
                      n369 = call "GetEnumFeatureEntryNum.vi"("handle"=w636, "pFeatureName"=w635, "error in (no error)"=w638) -> ("pEntryNum"=w641:u32, "error out"=w640:errorcluster)  [unwired: 7 in]
                      n370 = call "GetEnumFeatureEntrys.vi"("pFeatureName"=w635, "EntryNum"=w641, "handle"=w636, "error in (no error)"=w640) -> ("pLbEnumEntryList"=w643:string)  [unwired: 6 in, 1 out]
                      n371 = for {
                        N: w641 -> [_]
                        shift-right: [w655] -> _
                        shift-left: 0 ("offset past token") -> [w656]
                        shift-right: [w653] -> _
                        shift-left: w643 -> [w654]
                        shift-right: [w651] -> w632
                        shift-left: string[] [] -> [w652]
                        n372 = Scan String For Tokens(6:string[] [":"] ("delimiters (\\s,\\t,\\r,\\n)"), 8:w656, 9:w654) -> (1:w650:string, 2:w655:i32, 3:w653:string)  [unwired: 3 in, 1 out]
                        n373 = Build Array (concatenate)(w652, w650) -> (w651:string[])
                      }
                      n374 = local read "hIFDev"() -> (w642:i64)
                      n375 = call "GetEnumFeatureSymbol.vi"("pFeatureName"=w635, "handle"=w642) -> ("pEnumSymbol"=w631:string, "error out"=w639:errorcluster)  [unwired: 8 in]
                      n376 = while {
                        tunnel: w632 -> [w649]
                        tunnel: w631 -> [w647]
                        tunnel: [w645] -> w630
                        i -> [w645]
                        stop <- w646 stop-if-true
                        n377 = Index Array(array=w649, index=w645) -> (element=w648:string)
                        n378 = Equal?(x=w648, y=w647) -> (x = y?=w646:bool)
                      }
                      n379 = property on="DeviceScanType" class="Ring (strict)"(error in=w639, "Value"=w630) -> (error out=w634:errorcluster)  [unwired: 1 in, 1 out]
                      n380 = property on="DeviceScanType" class="Ring (strict)"(error in=w634, "Strings []"=w632) -> (error out=w633:errorcluster)  [unwired: 1 in, 1 out]
                    }
                  }
                }
                frame "ExposureTime" {
                  n381 = call "GetDoubleFeatureValue.vi"("pFeatureName"="ExposureTime", "handle"=w658, "error in (no error)"=w659) -> ("pDoubleValue"=w662:dbl, "error out"=w663:errorcluster)  [unwired: 7 in]
                  n382 = property on="ExposureTime" class="DigNum (strict)"(error in=w663, "Value"=w662) -> (error out=w661:errorcluster)  [unwired: 1 in, 1 out]
                }
                frame "GainRaw" {
                  n383 = call "GetDoubleFeatureValue.vi"("pFeatureName"="GainRaw", "handle"=w664, "error in (no error)"=w665) -> ("pDoubleValue"=w666:dbl, "error out"=w668:errorcluster)  [unwired: 7 in]
                  n384 = property on="GainRaw" class="DigNum (strict)"(error in=w668, "Value"=w666) -> (error out=w667:errorcluster)  [unwired: 1 in, 1 out]
                }
                frame "Width" {
                  n385 = call "GetIntFeatureValue.vi"("pFeatureName"="Width", "handle"=w670, "error in (no error)"=w671) -> ("pIntValue"=w673:i64, "error out"=w674:errorcluster)  [unwired: 7 in]
                  n386 = property on="Width" class="DigNum (strict)"(error in=w674, "Value"=w673) -> (error out=w672:errorcluster)  [unwired: 1 in, 1 out]
                }
                frame "Height" {
                  n387 = call "GetIntFeatureValue.vi"("pFeatureName"="Height", "handle"=w676, "error in (no error)"=w677) -> ("pIntValue"=w679:i64, "error out"=w680:errorcluster)  [unwired: 7 in]
                  n388 = property on="Height" class="DigNum (strict)"(error in=w680, "Value"=w679) -> (error out=w678:errorcluster)  [unwired: 1 in, 1 out]
                }
                frame "PixelFormat" {
                  w690 = "PixelFormat" ("pFeatureName")
                  n389 = call "GetEnumFeatureEntryNum.vi"("handle"=w682, "pFeatureName"=w690, "error in (no error)"=w696) -> ("pEntryNum"=w692:u32, "error out"=w695:errorcluster)  [unwired: 7 in]
                  n390 = call "GetEnumFeatureEntrys.vi"("pFeatureName"=w690, "EntryNum"=w692, "handle"=w682, "error in (no error)"=w695) -> ("pLbEnumEntryList"=w694:string, "error out"=w689:errorcluster)  [unwired: 6 in]
                  n391 = for {
                    N: w692 -> [_]
                    shift-right: [w707] -> _
                    shift-left: 0 ("offset past token") -> [w708]
                    shift-right: [w705] -> _
                    shift-left: w694 -> [w706]
                    shift-right: [w703] -> w684
                    shift-left: string[] [] -> [w704]
                    n392 = Scan String For Tokens(6:string[] [":"] ("delimiters (\\s,\\t,\\r,\\n)"), 8:w708, 9:w706) -> (1:w702:string, 2:w707:i32, 3:w705:string)  [unwired: 3 in, 1 out]
                    n393 = Build Array (concatenate)(w704, w702) -> (w703:string[])
                  }
                  n394 = property on="PixelFormat" class="Ring (strict)"(error in=w689, "Strings []"=w684) -> (error out=w688:errorcluster)  [unwired: 1 in, 1 out]
                  n395 = call "GetEnumFeatureSymbol.vi"("pFeatureName"=w690, "handle"=w682, "error in (no error)"=w688) -> ("pEnumSymbol"=w685:string, "error out"=w687:errorcluster)  [unwired: 7 in]
                  n396 = while {
                    tunnel: w684 -> [w701]
                    tunnel: w685 -> [w699]
                    tunnel: [w697] -> w683
                    i -> [w697]
                    stop <- w698 stop-if-true
                    n397 = Index Array(array=w701, index=w697) -> (element=w700:string)
                    n398 = Equal?(x=w700, y=w699) -> (x = y?=w698:bool)
                  }
                  n399 = property on="PixelFormat" class="Ring (strict)"(error in=w687, "Value"=w683) -> (error out=w686:errorcluster)  [unwired: 1 in, 1 out]
                }
                frame "TriggerSource" {
                  w715 = "TriggerSource" ("pFeatureName")
                  n400 = call "GetEnumFeatureEntryNum.vi"("handle"=w716, "pFeatureName"=w715, "error in (no error)"=w717) -> ("pEntryNum"=w721:u32, "error out"=w724:errorcluster)  [unwired: 7 in]
                  n401 = call "GetEnumFeatureEntrys.vi"("pFeatureName"=w715, "EntryNum"=w721, "handle"=w716, "error in (no error)"=w724) -> ("pLbEnumEntryList"=w723:string, "error out"=w719:errorcluster)  [unwired: 6 in]
                  n402 = for {
                    N: w721 -> [_]
                    shift-right: [w735] -> _
                    shift-left: 0 ("offset past token") -> [w736]
                    shift-right: [w733] -> _
                    shift-left: w723 -> [w734]
                    shift-right: [w731] -> w712
                    shift-left: string[] [] -> [w732]
                    n403 = Scan String For Tokens(6:string[] [":"] ("delimiters (\\s,\\t,\\r,\\n)"), 8:w736, 9:w734) -> (1:w730:string, 2:w735:i32, 3:w733:string)  [unwired: 3 in, 1 out]
                    n404 = Build Array (concatenate)(w732, w730) -> (w731:string[])
                  }
                  n405 = property on="TriggerSource" class="Ring (strict)"(error in=w719, "Strings []"=w712) -> (error out=w718:errorcluster)  [unwired: 1 in, 1 out]
                  n406 = call "GetEnumFeatureSymbol.vi"("pFeatureName"=w715, "handle"=w716, "error in (no error)"=w718) -> ("pEnumSymbol"=w711:string, "error out"=w714:errorcluster)  [unwired: 7 in]
                  n407 = while {
                    tunnel: w712 -> [w729]
                    tunnel: w711 -> [w727]
                    tunnel: [w725] -> w710
                    i -> [w725]
                    stop <- w726 stop-if-true
                    n408 = Index Array(array=w729, index=w725) -> (element=w728:string)
                    n409 = Equal?(x=w728, y=w727) -> (x = y?=w726:bool)
                  }
                  n410 = property on="TriggerSource" class="Ring (strict)"(error in=w714, "Value"=w710) -> (error out=w713:errorcluster)  [unwired: 1 in, 1 out]
                }
                frame "ExposureAuto" {
                  n411 = property on="DeviceInterfaceType" class="Ring (strict)"() -> ("Value"=w740:u16)  [unwired: 2 in, 2 out]
                  n412 = Not Equal?(x=w740, y=u16 3) -> (x != y?=w738:bool)
                  n413 = case shown="True" w738 {
                    tunnel: w743 -> [w745 w753]
                    tunnel: w742 -> [_ w752]
                    tunnel: [w744 w750] -> w741
                    frame False {
                      n414 = property on="ExposureAuto" class="Ring (strict)"(error in=w745, "DisabledEnum"=T6."Disabled and Grayed Out" ("Disabled")) -> (error out=w744:errorcluster)  [unwired: 1 in, 1 out]
                    }
                    frame True {
                      w761 = "ExposureAuto" ("pFeatureName")
                      n415 = call "GetEnumFeatureEntryNum.vi"("handle"=w752, "pFeatureName"=w761, "error in (no error)"=w753) -> ("pEntryNum"=w757:u32, "error out"=w754:errorcluster)  [unwired: 7 in]
                      n416 = call "GetEnumFeatureEntrys.vi"("pFeatureName"=w761, "EntryNum"=w757, "handle"=w752, "error in (no error)"=w754) -> ("pLbEnumEntryList"=w755:string, "error out"=w759:errorcluster)  [unwired: 6 in]
                      n417 = for {
                        N: w757 -> [_]
                        shift-right: [w772] -> _
                        shift-left: 0 ("offset past token") -> [w773]
                        shift-right: [w770] -> _
                        shift-left: w755 -> [w771]
                        shift-right: [w768] -> w749
                        shift-left: string[] [] -> [w769]
                        n418 = Scan String For Tokens(6:string[] [":"] ("delimiters (\\s,\\t,\\r,\\n)"), 8:w773, 9:w771) -> (1:w767:string, 2:w772:i32, 3:w770:string)  [unwired: 3 in, 1 out]
                        n419 = Build Array (concatenate)(w769, w767) -> (w768:string[])
                      }
                      n420 = property on="ExposureAuto" class="Ring (strict)"(error in=w759, "Strings []"=w749) -> (error out=w760:errorcluster)  [unwired: 1 in, 1 out]
                      n421 = call "GetEnumFeatureSymbol.vi"("pFeatureName"=w761, "handle"=w752, "error in (no error)"=w760) -> ("pEnumSymbol"=w748:string, "error out"=w751:errorcluster)  [unwired: 7 in]
                      n422 = while {
                        tunnel: w749 -> [w766]
                        tunnel: w748 -> [w764]
                        tunnel: [w762] -> w747
                        i -> [w762]
                        stop <- w763 stop-if-true
                        n423 = Index Array(array=w766, index=w762) -> (element=w765:string)
                        n424 = Equal?(x=w765, y=w764) -> (x = y?=w763:bool)
                      }
                      n425 = property on="ExposureAuto" class="Ring (strict)"(error in=w751, "Value"=w747) -> (error out=w750:errorcluster)  [unwired: 1 in, 1 out]
                    }
                  }
                }
              }
            }
            n426 = Merge Errors(w615) -> (w614:errorcluster)
          }
        }
      }
    }
    n427 = local read "QuitFlag"() -> (w588:bool)
    n428 = local write "error out"(w595) -> ()
  }
